vi "room catch recycle.vi"(8 "error in (no error)":errorcluster, 11 "Position in":T1) -> (0 "error out":errorcluster, 3 "Position out":T1)   [LabVIEW 2019]
uses:
  subVI/move/position cluster.ctl
  ctl/height.ctl
  ctl/servo act.ctl
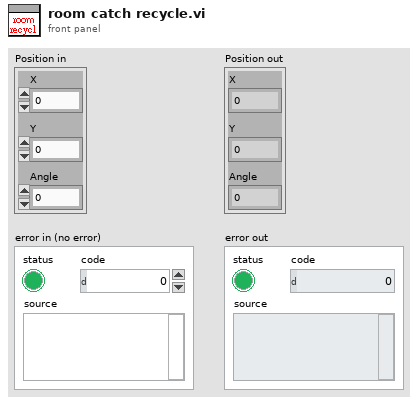
[diagram p1: front panel]
types:
  T1 = typedef "position cluster.ctl" = cluster{"X":dbl, "Y":dbl, "Angle":dbl}
  T2 = typedef "servo act.ctl" = enum16{"catch", "relax", "left idle", "center", "red relax", "left reg", "right reg"}
  T3 = typedef "height.ctl" = enum16{"IDLE", "recycle pre-catch", "recycle catch", "recycle zone", "vision height", "box 1", "box 2", "box 3", "box 1 pre", "box 2 pre", "box 3 pre", "reg 1", "reg 2", "reg 1 pre", "reg 2 pre", "put 1", "put 2", "put 3"}
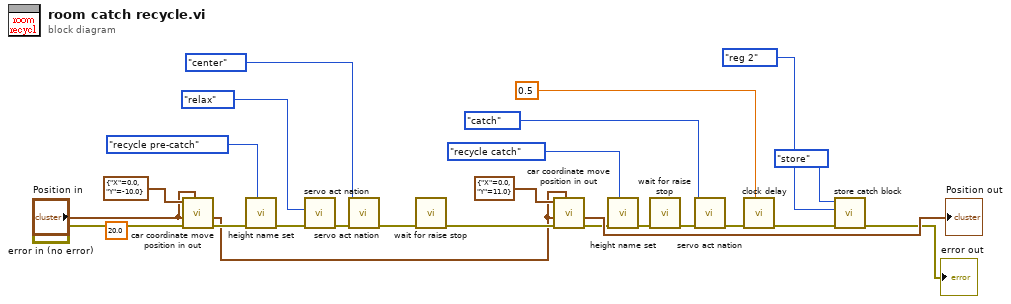
[diagram p0: block diagram]
diagram:
  (unwired) 20.0 ("speed")
  n1 = call "car coordinate move position in out.vi"("Position in 2"="Position in", "error in (no error)"="error in (no error)", "Position in"="Position in", "move"=cluster{"X":dbl, "Y":dbl} {"X"=0.0, "Y"=-10.0}) -> ("error out"=w11:errorcluster, "Position out"=w1:T1)  [unwired: 6 in]
  n2 = call "height name set.vi"("height name"=height."recycle pre-catch", "error in (no error)"=w11) -> ("error out"=w14:errorcluster)  [unwired: 9 in]
  n3 = call "servo act nation.vi"("error in"=w14, "servo act"=servo_act."relax") -> ("error out"=w15:errorcluster)  [unwired: 9 in]
  n4 = call "servo act nation.vi"("error in"=w15, "servo act"=servo_act."center") -> ("error out"=w3:errorcluster)  [unwired: 9 in]
  n5 = call "wait for raise stop.vi"("Error In"=w3) -> ("Error Out"=w4:errorcluster)  [unwired: 10 in]
  n6 = call "car coordinate move position in out.vi"("Position in 2"=w1, "error in (no error)"=w4, "Position in"=w1, "move"=cluster{"X":dbl, "Y":dbl} {"X"=0.0, "Y"=11.0}) -> ("error out"=w18:errorcluster, "Position out"=→"Position out":T1)  [unwired: 6 in]
  n7 = call "height name set.vi"("height name"=height."recycle catch", "error in (no error)"=w18) -> ("error out"=w20:errorcluster)  [unwired: 9 in]
  n8 = call "wait for raise stop.vi"("Error In"=w20) -> ("Error Out"=w21:errorcluster)  [unwired: 10 in]
  n9 = call "servo act nation.vi"("error in"=w21, "servo act"=servo_act."catch") -> ("error out"=w23:errorcluster)  [unwired: 9 in]
  n10 = call "clock delay.vi"("Delay Time (s)"=0.5, "error in (no error)"=w23) -> ("error out"=w8:errorcluster)  [unwired: 9 in]
  n11 = call "store catch block.vi"("error in"=w8, "reg"=enum16{"reg 1", "reg 2", "reg 3"}."reg 2", "store/catch"=enum16{"store", "catch out"}."store") -> ("error out"=→"error out":errorcluster)  [unwired: 8 in]
